vi "ICM Configuration Editor - Copy.vi"(11 "Inside a Program?":bool) -> ()   [LabVIEW 2018]
doc: "ICM Configuration Editor.vi\n\nThis Vi is a graphical configuration editor for ICM.\n\nInstrument Communication Module Version 1.0\nJuly, 2017 Original Code Consulting David Thomson\n www.originalcode.com"
uses:
  Controls/ICM Editor Tab.ctl
  Controls/ICM General Parameters.ctl
  Controls/ICM Config Editor State.ctl
  Controls/ICM Editor Command.ctl
  Scaling/Scaling Def.ctl
  Controls/ICM Config Command.ctl
  Query/Query.lvclass
  Scaling/Scaling.lvclass
  Scaling/Scaling.lvclass/Scaling.ctl
  Query/Query.lvclass/Query.ctl
  Query/Write Cycle Time (ms).vi
  Query/Read Cycle Time (ms).vi
  SubVIs/ICM Editor Stop.vi
  Parser/Parser.lvclass
panel:
  in  "Stop":bool
  in  "File Loaded?":bool
  out "Config File":path
  in  "Tab":T1
  in  "Save As":bool
  in  "Open/New":bool
  in  "Save":bool
  in  "Revert":bool
  in  "ICM General Parameters":T2 {"Time" format="%<%H:%M:%S>t"; "Date" format="%<%Y/%m/%d>T"; "Version" format="%.1g"}
  in  "Save Q":bool
  in  "Revert Q":bool
  in  "Cycle Time (ms)":u32
  in  "Queries":u16(ring) items=["Multiple Queries", "No Query", "Single Query"]
  in  "Bus":u16(ring) items=["Clock Time", "Modbus", "NI Analog", "Serial", "UDP"]
  in  "Parser":u16(ring) items=["General Parser", "Multi Sentence Parser", "No-op Parser", "Time Parser"]
  in  "Delete":bool
  in  "Add":bool
  in  "Instance":u16(ring) items=["(none)", "table", "hello"]
  in  "Save Scaling":bool
  in  "Revert Scaling":bool
  in  "Channel Scalings":i32(listbox)
  in  "Scaling":u16(ring) items=["Lookup Table", "Polynomial"]
  in  "Channel":u16(ring) items=["UTC Time", "Latitiude", "Longititude", "Course Over Ground", "UTS Date of Pos", "Magnetic Variation", "Hour", "Minute", "Second", "Lat", "Long", "Quality", "Satellites", "Horizontal Dilution", "Antenna Height", "Geoidal Height", "Fix Type", "PRN1", "PRN2", "PRN3", "PRN4", "PRN5", "PRN6", "PRN7", "PRN8", "PRN9", "PRN10", "PRN11", "PRN12", "Position Dilution", "Horizontal Dilution", "Vertical Dilution", "Satellites in View", "PRN 1", "Sat Elev 1", "Sat Az 1", "Signal to Noise 1", "PRN 2", "Sat Elev 2", "Sat Az 2", "Signal to Noise 2", "PRN 3", "Sat Elev 3", "Sat Az 3", "Signal to Noise 3", "PRN 4", "Sat Elev 4", "Sat Az 4", "Signal to Noise 4", "Satellites in View", "PRN 5", "Sat Elev 5", "Sat Az 5", "Signal to Noise 5", "PRN 6", "Sat Elev 6", "Sat Az 6", "Signal to Noise 6", "PRN 7", "Sat Elev 7", "Sat Az 7", "Signal to Noise 7", "PRN 8", "Sat Elev 8", "Sat Az 8", "Signal to Noise 8", "Total Number of Satellites", "PRN 9", "Sat Elev 9", "Sat Az 9", "Signal to Noise 9", "PRN 10", "Sat Elev 10", "Sat Az 10", "Signal to Noise 10", "PRN 11", "Sat Elev 11", "Sat Az 11", "Signal to Noise 11", "PRN 12", "Sat Elev 12", "Sat Az 12", "Signal to Noise 12"]
  in  "Output":u16(ring) items=["NI Digital Out"]
  out "Error":errorcluster
  in  "Error Continue":bool
  in  "Error Quit":bool
  in  "Initializer":u16(ring) items=["No Init", "String Init"]
  # "The values for these\nparameters are generally\nset by the ICM system and\nneed not be edited directly."
  # "Entries surrounded by \"***\" are present in the configuration file but\ndo not correspond to existing Channels, Scalings, or Instances."
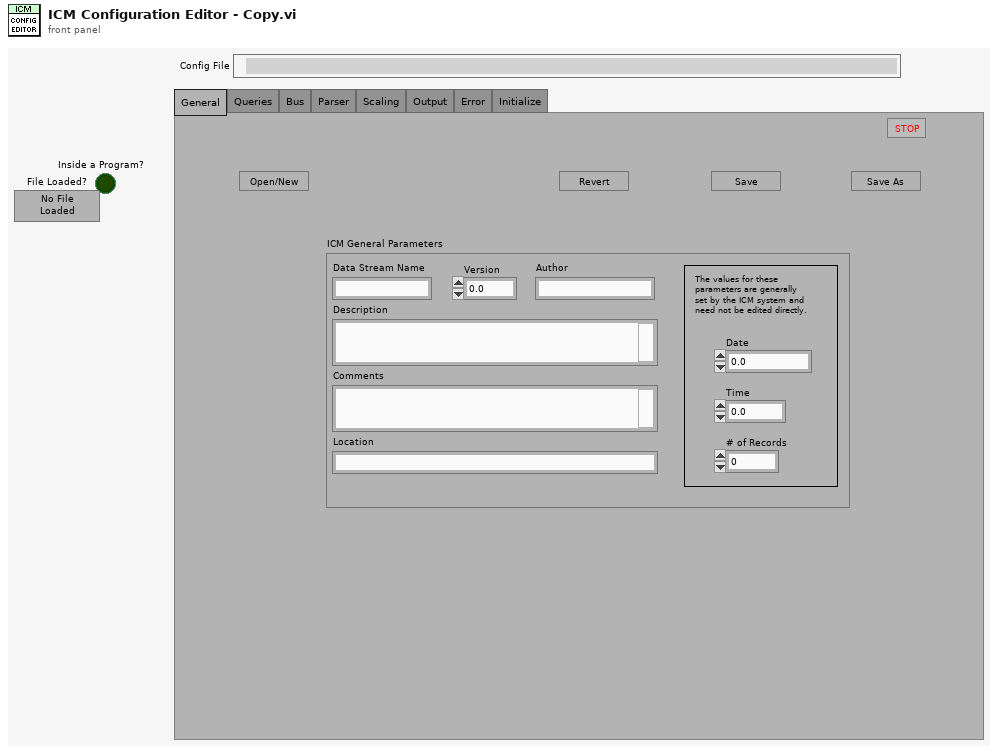
[diagram p1: front panel]
types:
  T1 = typedef "ICM Editor Tab.ctl" = enum32{"General", "Queries", "Bus", "Parser", "Scaling", "Output", "Error", "Initialize"}
  T2 = typedef "ICM General Parameters.ctl" = cluster{"Data Stream Name":string, "Version":sgl, "Author":string, "Description":string, "Comments":string, "Date":dbl, "Time":dbl, "Location":string, "# of Records":i32}
  T3 = typedef "ICM Config Editor State.ctl" = enum16{"Init", "Wait", "Read", "Write", "Load Queries", "Load Bus", "Load Parser", "Display Scaling", "Load Output", "Load Initializer", "Error", "Stop"}
  T4 = typedef "ICM Editor Command.ctl" = enum16{"No-op", "Exit"}
  T5 = typedef "ICM Config Command.ctl" = enum16{"No-op", "Re-Display Sc."}
  T6 = enum8{"Enabled", "Disabled", "Disabled and Grayed Out"}
  T7 = enum32{"Page Enabled", "Page Disabled", "Page Disabled & Grayed"}
  T8 = typedef "Scaling Def.ctl" = cluster{"Channel":string, "Scaling":string, "Instance":string}
  T9 = cluster{"Query.lvclass":refnum<class "Query.lvclass">, "ICM General Parameters":T2, "Output Queue":refnum<queue>, "Init Queue":refnum<queue>, "Config Queue":refnum<queue>, "Scaling Queue":refnum<queue>, "Query Queue":refnum<queue>, "Parser Queue":refnum<queue>, "Bus Queue":refnum<queue>, "Queries Loaded":bool, "Bus Loaded":bool, "Parser Loaded":bool, "Init Loaded":bool, "Output Loaded":bool, "Scaling Loaded":i32, "Instance Loaded":i32, "Scalings":T8[], "Flash?":bool}
  T10 = cluster{"RingText.Text":string, "RingText.Text":string, "RingText.Text":string}
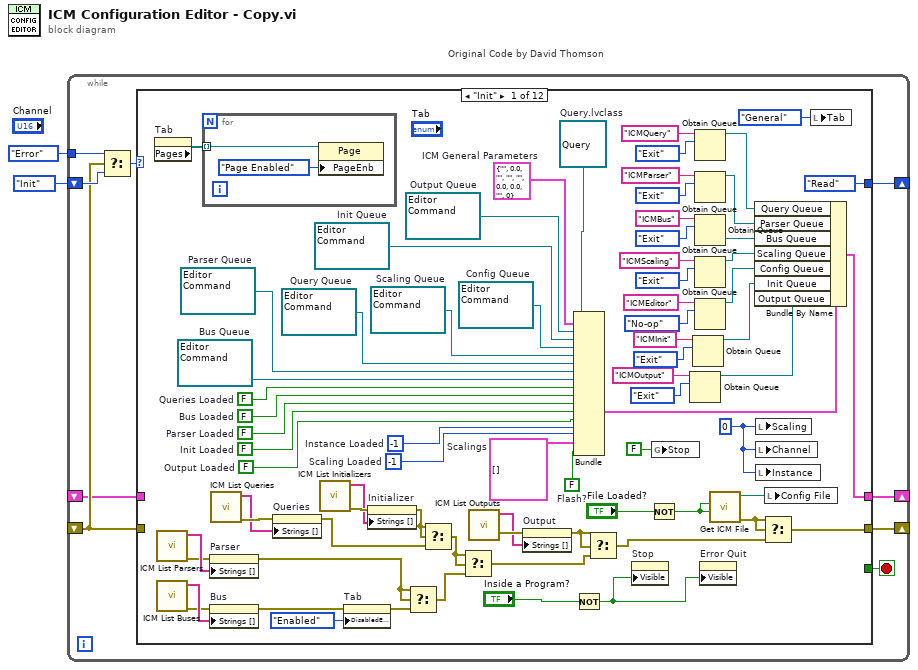
[diagram p0: block diagram]
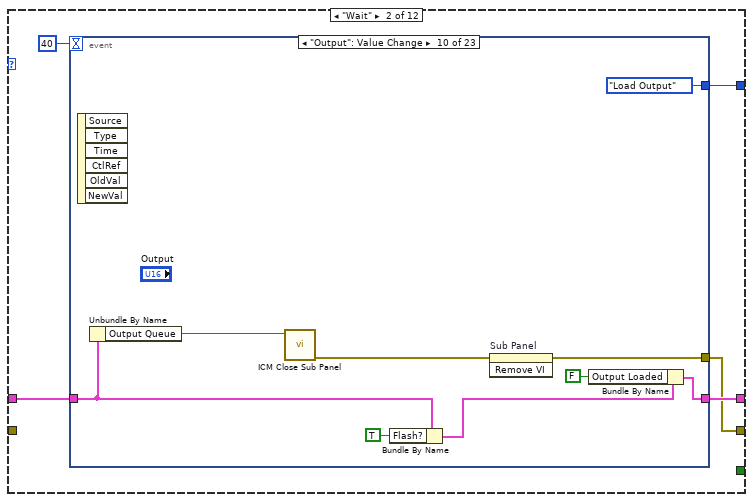
[diagram p2: hidden frame]
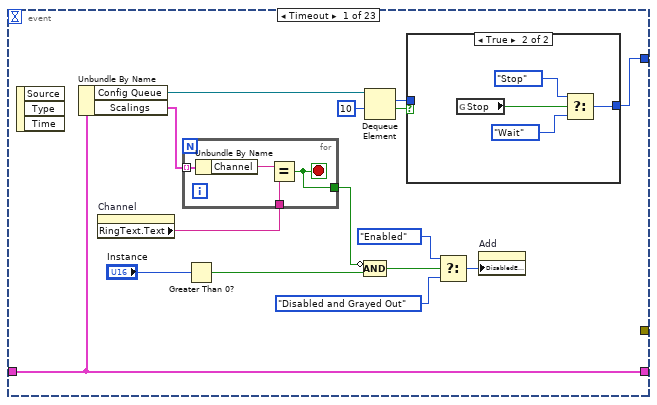
[diagram p3: hidden frame]
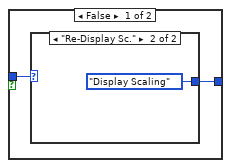
[diagram p4: hidden frame]
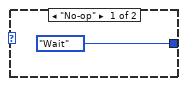
[diagram p5: hidden frame]
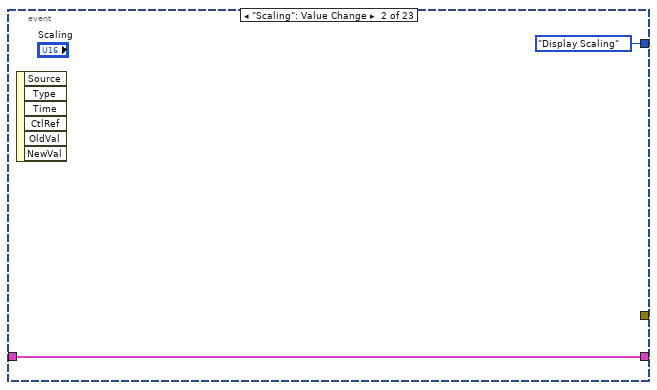
[diagram p6: hidden frame]
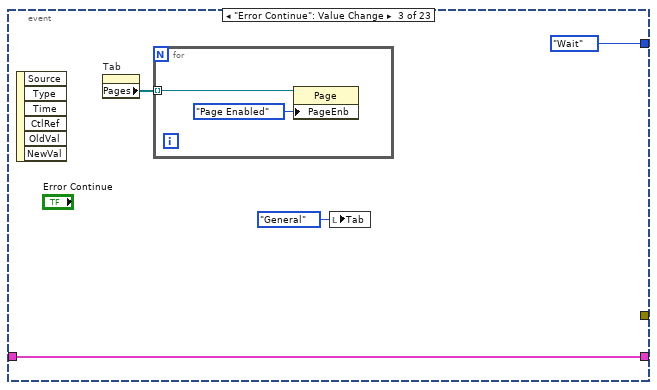
[diagram p7: hidden frame]
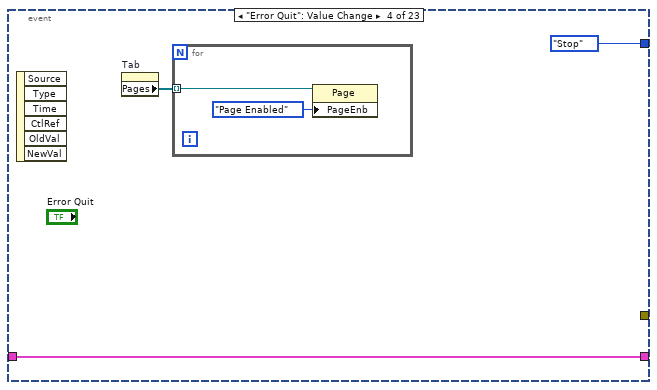
[diagram p8: hidden frame]
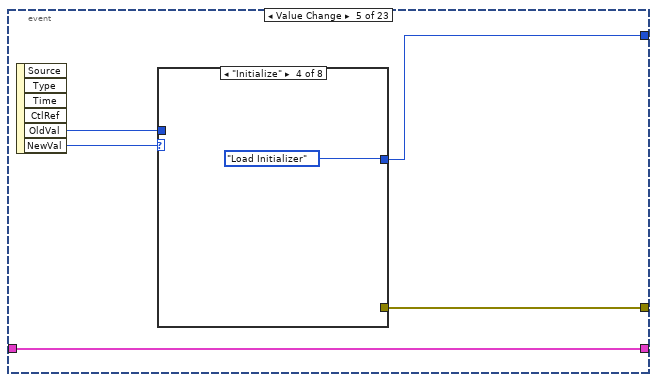
[diagram p9: hidden frame]
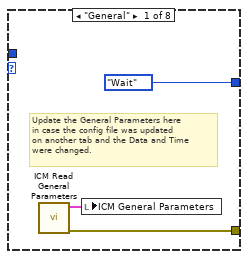
[diagram p10: hidden frame]
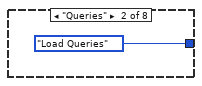
[diagram p11: hidden frame]
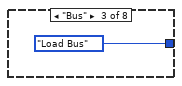
[diagram p12: hidden frame]
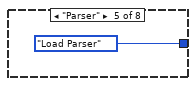
[diagram p13: hidden frame]
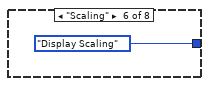
[diagram p14: hidden frame]
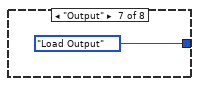
[diagram p15: hidden frame]
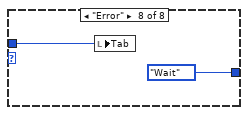
[diagram p16: hidden frame]
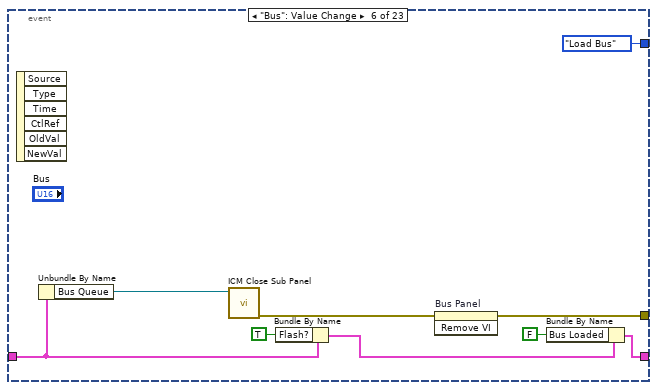
[diagram p17: hidden frame]
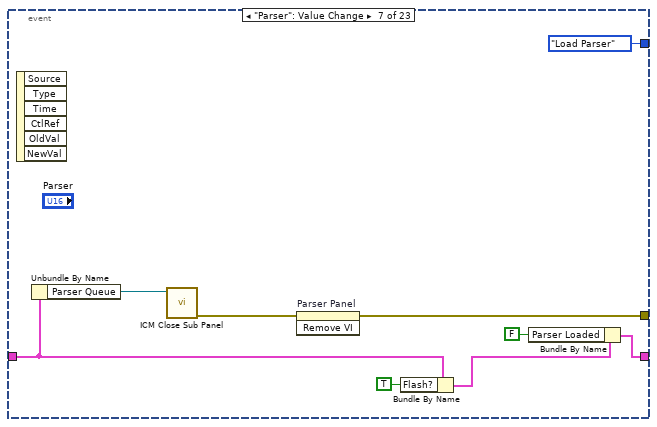
[diagram p18: hidden frame]
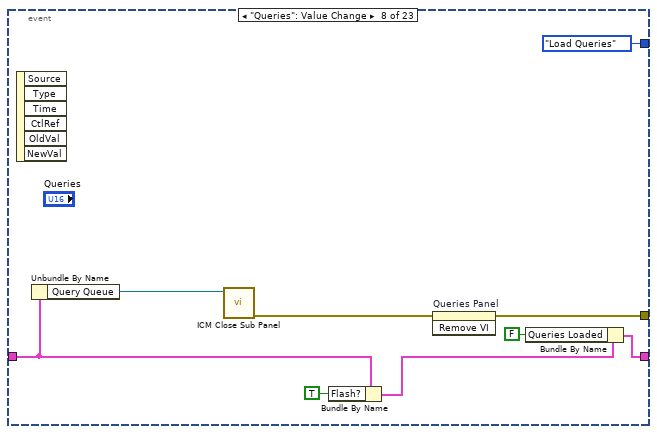
[diagram p19: hidden frame]
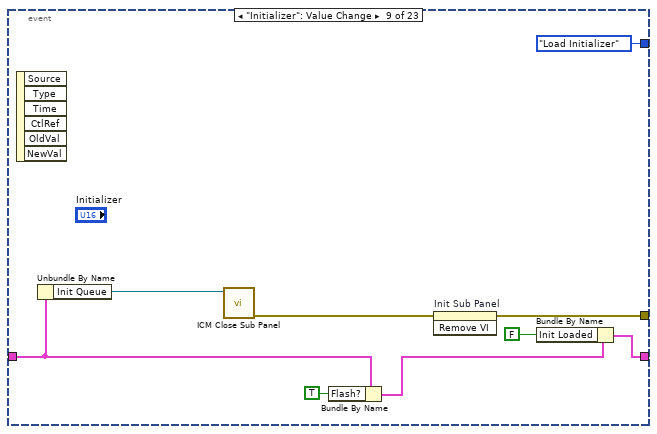
[diagram p20: hidden frame]
diagram:
  n1 = while "Original Code by David Thomson" {
    shift-right: [w5] -> _
    shift-left: ICM_Config_Editor_State."Init" ("Config State") -> [w9]
    shift-right: [w10] -> _
    shift-left: _ -> [w6]
    tunnel: ICM_Config_Editor_State."Error" ("Config State") -> [w7]
    shift-right: [w4] -> _
    shift-left: _ -> [w3]
    stop <- w11 stop-if-true
    n2 = Select(t=w7, s=w6, f=w9) -> (s? t:f=w8:T3)
    n3 = case shown="\"Init\"" w8 {
      tunnel: [_ _ _ _ _ _ _ _ _ _ _ TRUE] -> w11
      tunnel: [w78 w88 w298 w325 w334 w369 w398 w430 w481 _ _ _] -> w10
      tunnel: w6 -> [_ _ _ _ _ _ _ _ _ _ w554 _]
      tunnel: [ICM_Config_Editor_State."Read" ("Config State") w91 ICM_Config_Editor_State."Wait" ("Config State") ICM_Config_Editor_State."Wait" ("Config State") ICM_Config_Editor_State."Wait" ("Config State") ICM_Config_Editor_State."Wait" ("Config State") ICM_Config_Editor_State."Write" ("Config State") ICM_Config_Editor_State."Write" ("Config State") ICM_Config_Editor_State."Wait" ("Config State") ICM_Config_Editor_State."Wait" ("Config State") ICM_Config_Editor_State."Wait" ("Config State") ICM_Config_Editor_State."Stop" ("Config State")] -> w5
      tunnel: [w71 w89 w314 w328 w330 w366 w399 w431 w480 w520 w550 w583] -> w4
      tunnel: w3 -> [_ w90 w316 w328 w336 w367 w400 w432 w467 w520 w550 w583]
      frame "Init" {
        w17 = FALSE  # Output Loaded
        w21 = refnum<queue> refnum items=["No-op", "Exit"]  # Output Queue
        w22 = refnum<queue> refnum items=["No-op", "Exit"]  # Init Queue
        w32 = FALSE  # Init Loaded
        w33 = FALSE  # Flash?
        w42 = refnum<class "Query.lvclass"> refnum  # Query.lvclass
        w31 = refnum<queue> refnum items=["No-op", "Re-Display Sc."]  # Config Queue
        w48 = refnum<queue> refnum items=["No-op", "Exit"]  # Scaling Queue
        w51 = u16 0
        w52 = -1  # Instance Loaded
        w54 = -1  # Scaling Loaded
        w53 = T8[] []  # Scalings
        w59 = refnum<queue> refnum items=["No-op", "Exit"]  # Query Queue
        w67 = refnum<queue> refnum items=["No-op", "Exit"]  # Parser Queue
        w68 = FALSE  # Parser Loaded
        w69 = FALSE  # Bus Loaded
        w70 = FALSE  # Queries Loaded
        w74 = refnum<queue> refnum items=["No-op", "Exit"]  # Bus Queue
        w44 = T2 {"Data Stream Name"="", "Version"=0.0, "Author"="", "Description"="", "Comments"="", "Date"=0.0, "Time"=0.0, "Location"="", "# of Records"=0}  # ICM General Parameters
        n4 = property on="Tab" class="TabCtl (strict)"() -> ("Pages"=w77:refnum<vi>[])  [unwired: 2 in, 2 out]
        n5 = call "ICM List Parsers.vi"() -> ("error out"=w63:errorcluster, "Parsers"=w64:string[])  [unwired: 10 in]
        n6 = call "ICM List Buses.vi"() -> ("error out"=w84:errorcluster, "Buses"=w85:string[])  [unwired: 10 in]
        n7 = for {
          tunnel: w77 -> [w87] mode=indexing
          n8 = property class="Page"(reference=w87, "PageEnb"=T7."Page Enabled" ("Page Enabled State")) -> ()  [unwired: 1 in, 2 out]
        }
        n9 = property on="Parser" class="Ring (strict)"(error in=w63, "Strings []"=w64) -> (error out=w61:errorcluster)  [unwired: 1 in, 1 out]
        n10 = property on="Bus" class="Ring (strict)"(error in=w84, "Strings []"=w85) -> (error out=w82:errorcluster)  [unwired: 1 in, 1 out]
        n11 = call "ICM List Queries.vi"() -> ("error out"=w57:errorcluster, "Queries"=w56:string[])  [unwired: 10 in]
        n12 = property on="Queries" class="Ring (strict)"(error in=w57, "Strings []"=w56) -> (error out=w27:errorcluster)  [unwired: 1 in, 1 out]
        n13 = call "ICM List Initializers.vi"() -> ("error out"=w26:errorcluster, "Initializers"=w25:string[])  [unwired: 10 in]
        n14 = property on="Tab" class="TabCtl (strict)"(error in=w82, "DisabledEnum"=T6."Enabled" ("Disabled")) -> (error out=w62:errorcluster)  [unwired: 1 in, 1 out]
        n15 = property on="Initializer" class="Ring (strict)"(error in=w26, "Strings []"=w25) -> (error out=w24:errorcluster)  [unwired: 1 in, 1 out]
        n16 = Select(t=w61, s=w61, f=w62) -> (s? t:f=w55:errorcluster)
        n17 = Select(t=w24, s=w24, f=w27) -> (s? t:f=w28:errorcluster)
        n18 = Select(t=w28, s=w28, f=w55) -> (s? t:f=w13:errorcluster)
        n19 = call "ICM List Outputs.vi"() -> ("error out"=w16:errorcluster, "Initializers"=w15:string[])  [unwired: 10 in]
        n20 = property on="Output" class="Ring (strict)"(error in=w16, "Strings []"=w15) -> (error out=w12:errorcluster)  [unwired: 1 in, 1 out]
        n21 = Bundle("Query.lvclass"=w42, "ICM General Parameters"=w44, "Output Queue"=w21, "Init Queue"=w22, "Config Queue"=w31, "Scaling Queue"=w48, "Query Queue"=w59, "Parser Queue"=w67, "Bus Queue"=w74, "Queries Loaded"=w70, "Bus Loaded"=w69, "Parser Loaded"=w68, "Init Loaded"=w32, "Output Loaded"=w17, "Scaling Loaded"=w54, "Instance Loaded"=w52, "Scalings"=w53, "Flash?"=w33) -> (w73:T9)  [unwired: 1 in]
        n22 = Not(x="Inside a Program?") -> (.not. x?=w35:bool)
        n23 = Select(t=w12, s=w12, f=w13) -> (s? t:f=w14:errorcluster)
        n24 = property on="Stop" class="Bool"("Visible"=w35) -> ()  [unwired: 2 in, 2 out]
        n25 = Not(x="File Loaded?") -> (.not. x?=w37:bool)
        n26 = global write "ICM Editor Stop.vi" "Stop"(FALSE ("Stop")) -> ()
        n27 = Obtain Queue(name (unnamed)="ICMOutput", element data type=ICM_Editor_Command."Exit" ("Editor Command")) -> (queue out=w18:refnum<queue>)  [unwired: 3 in, 2 out]
        n28 = Obtain Queue(name (unnamed)="ICMInit", element data type=ICM_Editor_Command."Exit" ("Editor Command")) -> (queue out=w23:refnum<queue>)  [unwired: 3 in, 2 out]
        n29 = Obtain Queue(name (unnamed)="ICMQuery", element data type=ICM_Editor_Command."Exit" ("Editor Command")) -> (queue out=w58:refnum<queue>)  [unwired: 3 in, 2 out]
        n30 = Obtain Queue(name (unnamed)="ICMParser", element data type=ICM_Editor_Command."Exit" ("Editor Command")) -> (queue out=w65:refnum<queue>)  [unwired: 3 in, 2 out]
        n31 = Obtain Queue(name (unnamed)="ICMBus", element data type=ICM_Editor_Command."Exit" ("Editor Command")) -> (queue out=w72:refnum<queue>)  [unwired: 3 in, 2 out]
        n32 = Obtain Queue(name (unnamed)="ICMScaling", element data type=ICM_Editor_Command."Exit" ("Editor Command")) -> (queue out=w47:refnum<queue>)  [unwired: 3 in, 2 out]
        n33 = Obtain Queue(name (unnamed)="ICMEditor", element data type=ICM_Config_Command."No-op" ("Editor Command")) -> (queue out=w43:refnum<queue>)  [unwired: 3 in, 2 out]
        n34 = property on="Error Quit" class="Bool"("Visible"=w35) -> ()  [unwired: 2 in, 2 out]
        n35 = call "Get ICM File.vi"("Re-Init?"=w37, "Allow New?"=w37) -> ("error out"=w79:errorcluster, "ICM File"=w76:path)  [unwired: 8 in]
        n36 = Bundle By Name(cluster=w73, "Query Queue"=w58, "Parser Queue"=w65, "Bus Queue"=w72, "Scaling Queue"=w47, "Config Queue"=w43, "Init Queue"=w23, "Output Queue"=w18) -> (w71:T9)
        n37 = local write "Scaling"(w51) -> ()
        n38 = local write "Channel"(w51) -> ()
        n39 = local write "Instance"(w51) -> ()
        n40 = Select(t=w79, s=w79, f=w14) -> (s? t:f=w78:errorcluster)
        n41 = local write "Config File"(w76) -> ()
        n42 = local write "Tab"(ICM_Editor_Tab."General" ("Tab")) -> ()
      }
      frame "Wait" {
        n43 = event shown="[9] \"Output\": Value Change" {
          selector: _ -> [_ _ _ _ _ _ _ _ _ _ _ _ _ _ _ _ _ _ _ _ _ _ _]
          dyn-events: _ -> [_ _ _ _ _ _ _ _ _ _ _ _ _ _ _ _ _ _ _ _ _ _ _]
          timeout: 40 -> [_ _ _ _ _ _ _ _ _ _ _ _ _ _ _ _ _ _ _ _ _ _ _]
          tunnel: [w103 ICM_Config_Editor_State."Display Scaling" ("Config State") ICM_Config_Editor_State."Wait" ("Config State") ICM_Config_Editor_State."Stop" ("Config State") w136 ICM_Config_Editor_State."Load Bus" ("Config State") ICM_Config_Editor_State."Load Parser" ("Config State") ICM_Config_Editor_State."Load Queries" ("Config State") ICM_Config_Editor_State."Load Initializer" ("Config State") ICM_Config_Editor_State."Load Output" ("Config State") ICM_Config_Editor_State."Wait" ("Config State") ICM_Config_Editor_State."Wait" ("Config State") ICM_Config_Editor_State."Write" ("Config State") ICM_Config_Editor_State."Read" ("Config State") w223 ICM_Config_Editor_State."Stop" ("Config State") ICM_Config_Editor_State."Display Scaling" ("Config State") ICM_Config_Editor_State."Display Scaling" ("Config State") ICM_Config_Editor_State."Wait" ("Config State") ICM_Config_Editor_State."Display Scaling" ("Config State") ICM_Config_Editor_State."Wait" ("Config State") ICM_Config_Editor_State."Wait" ("Config State") ICM_Config_Editor_State."Wait" ("Config State")] -> w91
          tunnel: w90 -> [w107 w121 w122 w128 w135 w150 w158 w167 w178 w187 w194 w198 w203 w208 w214 w237 w243 w259 w268 w273 w280 w289 w292]
          tunnel: [w107 w121 w122 w128 w135 w155 w165 w174 w183 w192 w194 w198 w201 w208 w222 w237 w242 w258 w268 w272 w280 w289 w292] -> w89
          tunnel: [_ _ _ _ w134 w156 w163 w172 w177 w185 _ _ _ _ w213 _ _ _ w264 w271 _ w284 w290] -> w88
          event Timeout {
            n44 = event-data() -> ()  [unwired: 1 in, 3 out]
            n45 = Unbundle By Name(w107) -> ("Config Queue"=w106:refnum<queue>, "Scalings"=w101:T8[])
            n46 = property on="Channel" class="Ring (strict)"() -> ("RingText.Text"=w100:string)  [unwired: 2 in, 2 out]
            n47 = for {
              tunnel: w101 -> [w109] mode=indexing
              tunnel: [w111] -> w99
              tunnel: w100 -> [w108]
              stop <- w111 stop-if-true
              n48 = Unbundle By Name(w109) -> ("Channel"=w110:string)
              n49 = Equal?(x=w110, y=w108) -> (x = y?=w111:bool)
            }
            n50 = Greater Than 0?(x="Instance") -> (x > 0?=w97:bool)
            n51 = Compound Arithmetic op=AND(invert w99, w97) -> (w94:bool)
            n52 = Dequeue Element(queue=w106, timeout in ms (-1)=10) -> (element=w102:T5, timed out?=w104:bool)  [unwired: 1 in, 2 out]
            n53 = case shown="True" w104 {
              tunnel: [w112 w119] -> w103
              tunnel: w102 -> [w113 _]
              frame False {
                n54 = case shown="\"Re-Display Sc.\"" w113 {
                  tunnel: [ICM_Config_Editor_State."Wait" ("Config State") ICM_Config_Editor_State."Display Scaling" ("Config State")] -> w112
                  frame "No-op" {
                  }
                  frame "Re-Display Sc." {
                  }
                }
              }
              frame True {
                n55 = global read "ICM Editor Stop.vi" "Stop"() -> (w118:bool)
                n56 = Select(t=ICM_Config_Editor_State."Stop" ("Config State"), s=w118, f=ICM_Config_Editor_State."Wait" ("Config State")) -> (s? t:f=w119:T3)
              }
            }
            n57 = Select(t=T6."Enabled" ("Disabled"), s=w94, f=T6."Disabled and Grayed Out" ("Disabled")) -> (s? t:f=w93:T6)
            n58 = property on="Add" class="Bool"("DisabledEnum"=w93) -> ()  [unwired: 2 in, 2 out]
          }
          event "Scaling": Value Change {
            n59 = event-data() -> ()  [unwired: 1 in, 6 out]
          }
          event "Error Continue": Value Change {
            n60 = event-data() -> ()  [unwired: 1 in, 6 out]
            n61 = property on="Tab" class="TabCtl (strict)"() -> ("Pages"=w123:refnum<vi>[])  [unwired: 2 in, 2 out]
            n62 = for {
              tunnel: w123 -> [w127] mode=indexing
              n63 = property class="Page"(reference=w127, "PageEnb"=T7."Page Enabled" ("Page Enabled State")) -> ()  [unwired: 1 in, 2 out]
            }
            n64 = local write "Tab"(ICM_Editor_Tab."General" ("Tab")) -> ()
          }
          event "Error Quit": Value Change {
            n65 = event-data() -> ()  [unwired: 1 in, 6 out]
            n66 = property on="Tab" class="TabCtl (strict)"() -> ("Pages"=w129:refnum<vi>[])  [unwired: 2 in, 2 out]
            n67 = for {
              tunnel: w129 -> [w132] mode=indexing
              n68 = property class="Page"(reference=w132, "PageEnb"=T7."Page Enabled" ("Page Enabled State")) -> ()  [unwired: 1 in, 2 out]
            }
          }
          event Value Change {
            n69 = event-data() -> ("OldVal"=w133:T1, "NewVal"=w137:T1)  [unwired: 1 in, 4 out]
            n70 = case shown="\"Initialize\"" w137 {
              tunnel: [ICM_Config_Editor_State."Wait" ("Config State") ICM_Config_Editor_State."Load Queries" ("Config State") ICM_Config_Editor_State."Load Bus" ("Config State") ICM_Config_Editor_State."Load Initializer" ("Config State") ICM_Config_Editor_State."Load Parser" ("Config State") ICM_Config_Editor_State."Display Scaling" ("Config State") ICM_Config_Editor_State."Load Output" ("Config State") ICM_Config_Editor_State."Wait" ("Config State")] -> w136
              tunnel: [w138 _ _ _ _ _ _ _] -> w134
              tunnel: w133 -> [_ _ _ _ _ _ _ w147]
              frame "General" {
                # "Update the General Parameters here\nin case the config file was updated\non another tab and the Data and Time\nwere changed."
                n71 = call "ICM Read General Parameters.vi"() -> ("error out"=w138:errorcluster, "ICM General Parameters"=w139:T2)  [unwired: 7 in, 3 out]
                n72 = local write "ICM General Parameters"(w139) -> ()
              }
              frame "Queries" {
              }
              frame "Bus" {
              }
              frame "Initialize" {
              }
              frame "Parser" {
              }
              frame "Scaling" {
              }
              frame "Output" {
              }
              frame "Error" {
                n73 = local write "Tab"(w147) -> ()
              }
            }
          }
          event "Bus": Value Change {
            n74 = event-data() -> ()  [unwired: 1 in, 6 out]
            n75 = Unbundle By Name(w150) -> ("Bus Queue"=w153:refnum<queue>)
            n76 = call "ICM Close Sub Panel.vi"("Queue"=w153) -> ("error out"=w152:errorcluster)  [unwired: 9 in, 1 out]
            n77 = Bundle By Name(cluster=w150, "Flash?"=TRUE) -> (w151:T9)
            n78 = invoke on="Bus Panel" class="SubPnl" method="Remove VI"(error in=w152) -> (error out=w156:errorcluster)  [unwired: 2 in, 2 out]
            n79 = Bundle By Name(cluster=w151, "Bus Loaded"=FALSE) -> (w155:T9)
          }
          event "Parser": Value Change {
            n80 = event-data() -> ()  [unwired: 1 in, 6 out]
            n81 = Unbundle By Name(w158) -> ("Parser Queue"=w162:refnum<queue>)
            n82 = call "ICM Close Sub Panel.vi"("Queue"=w162) -> ("error out"=w161:errorcluster)  [unwired: 9 in, 1 out]
            n83 = invoke on="Parser Panel" class="SubPnl" method="Remove VI"(error in=w161) -> (error out=w163:errorcluster)  [unwired: 2 in, 2 out]
            n84 = Bundle By Name(cluster=w158, "Flash?"=TRUE) -> (w159:T9)
            n85 = Bundle By Name(cluster=w159, "Parser Loaded"=FALSE ("Bus Loaded")) -> (w165:T9)
          }
          event "Queries": Value Change {
            n86 = event-data() -> ()  [unwired: 1 in, 6 out]
            n87 = Unbundle By Name(w167) -> ("Query Queue"=w171:refnum<queue>)
            n88 = call "ICM Close Sub Panel.vi"("Queue"=w171) -> ("error out"=w170:errorcluster)  [unwired: 9 in, 1 out]
            n89 = Bundle By Name(cluster=w167, "Flash?"=TRUE) -> (w168:T9)
            n90 = invoke on="Queries Panel" class="SubPnl" method="Remove VI"(error in=w170) -> (error out=w172:errorcluster)  [unwired: 2 in, 2 out]
            n91 = Bundle By Name(cluster=w168, "Queries Loaded"=FALSE ("Bus Loaded")) -> (w174:T9)
          }
          event "Initializer": Value Change {
            n92 = event-data() -> ()  [unwired: 1 in, 6 out]
            n93 = Unbundle By Name(w178) -> ("Init Queue"=w181:refnum<queue>)
            n94 = call "ICM Close Sub Panel.vi"("Queue"=w181) -> ("error out"=w176:errorcluster)  [unwired: 9 in, 1 out]
            n95 = Bundle By Name(cluster=w178, "Flash?"=TRUE) -> (w179:T9)
            n96 = invoke on="Init Sub Panel" class="SubPnl" method="Remove VI"(error in=w176) -> (error out=w177:errorcluster)  [unwired: 2 in, 2 out]
            n97 = Bundle By Name(cluster=w179, "Init Loaded"=FALSE ("Bus Loaded")) -> (w183:T9)
          }
          event "Output": Value Change {
            n98 = event-data() -> ()  [unwired: 1 in, 6 out]
            n99 = Unbundle By Name(w187) -> ("Output Queue"=w190:refnum<queue>)
            n100 = call "ICM Close Sub Panel.vi"("Queue"=w190) -> ("error out"=w186:errorcluster)  [unwired: 9 in, 1 out]
            n101 = Bundle By Name(cluster=w187, "Flash?"=TRUE) -> (w188:T9)
            n102 = invoke on="Sub Panel" class="SubPnl" method="Remove VI"(error in=w186) -> (error out=w185:errorcluster)  [unwired: 2 in, 2 out]
            n103 = Bundle By Name(cluster=w188, "Output Loaded"=FALSE ("Bus Loaded")) -> (w192:T9)
          }
          event Value Change {
            w196 = TRUE ("Blinking")
            n104 = event-data() -> ()  [unwired: 1 in, 6 out]
            n105 = property on="Revert" class="Bool"("Blinking"=w196) -> ()  [unwired: 2 in, 2 out]
            n106 = property on="Save" class="Bool"("Blinking"=w196) -> ()  [unwired: 2 in, 2 out]
          }
          event "Revert": Value Change {
            w200 = FALSE ("Blinking")
            n107 = event-data() -> ()  [unwired: 1 in, 6 out]
            n108 = Unbundle By Name(w198) -> ("ICM General Parameters"=w197:T2)
            n109 = local write "ICM General Parameters"(w197) -> ()
            n110 = property on="Revert" class="Bool"("Blinking"=w200) -> ()  [unwired: 2 in, 2 out]
            n111 = property on="Save" class="Bool"("Blinking"=w200) -> ()  [unwired: 2 in, 2 out]
          }
          event "Save": Value Change {
            w205 = FALSE ("Blinking")
            n112 = event-data() -> ()  [unwired: 1 in, 6 out]
            n113 = property on="Revert" class="Bool"("Blinking"=w205) -> ()  [unwired: 2 in, 2 out]
            n114 = property on="Save" class="Bool"("Blinking"=w205) -> ()  [unwired: 2 in, 2 out]
            n115 = Bundle By Name(cluster=w203, "ICM General Parameters"="ICM General Parameters") -> (w201:T9)
          }
          event "Open/New": Value Change {
            w206 = TRUE ("Re-Init?")
            n116 = event-data() -> ()  [unwired: 1 in, 6 out]
            n117 = call "Get ICM File.vi"("Re-Init?"=w206, "Allow New?"=w206) -> ("ICM File"=→"Config File":path)  [unwired: 8 in, 1 out]
          }
          event "Save As": Value Change {
            n118 = event-data() -> ()  [unwired: 1 in, 6 out]
            n119 = call "Get ICM File.vi"() -> ("error out"=w216:errorcluster, "ICM File"=w215:path)  [unwired: 10 in]
            n120 = Strip Path(path=w215) -> (stripped path=w221:path)  [unwired: 1 out]
            n121 = call "File Dialog"("start path"=w221, "prompt"="Name the new configuration file:" ("pattern label"), "error in"=w216, "pattern (all files)"=".icm", "pattern label"="ICM Configuraiton File") -> ("selected path"=w217:path, "cancelled"=w211:bool, "error out"=w212:errorcluster)  [unwired: 7 in, 1 out]
            n122 = Compound Arithmetic op=AND(invert w211, invert w212) -> (w210:bool)
            n123 = case shown="True" w210 {
              tunnel: [ICM_Config_Editor_State."Wait" ("Config State") ICM_Config_Editor_State."Write" ("Config State")] -> w223
              tunnel: [w225 w227] -> w222
              tunnel: w217 -> [_ w232]
              tunnel: w215 -> [_ w234]
              tunnel: w214 -> [w225 w228]
              tunnel: [_ w229] -> w213
              frame False {
              }
              frame True {
                w235 = FALSE ("Blinking")
                n124 = Copy(9:TRUE ("overwrite (F)"), 10:w232, 11:w234) -> (0:w230:errorcluster)  [unwired: 2 in, 2 out]
                n125 = call "Get ICM File.vi"("ICM File In"=w232) -> ("error out"=w231:errorcluster)  [unwired: 9 in, 1 out]
                n126 = Select(t=w231, s=w231, f=w230) -> (s? t:f=w229:errorcluster)
                n127 = local read "ICM General Parameters"() -> (w226:T2)
                n128 = Bundle By Name(cluster=w228, "ICM General Parameters"=w226) -> (w227:T9)
                n129 = property on="Revert" class="Bool"("Blinking"=w235) -> ()  [unwired: 2 in, 2 out]
                n130 = property on="Save" class="Bool"("Blinking"=w235) -> ()  [unwired: 2 in, 2 out]
              }
            }
          }
          event "Stop": Value Change {
            n131 = event-data() -> ()  [unwired: 1 in, 6 out]
          }
          event "Add": Value Change {
            n132 = event-data() -> ()  [unwired: 1 in, 6 out]
            n133 = property on="Channel" class="Ring (strict)"() -> ("RingText.Text"=w241:string)  [unwired: 2 in, 2 out]
            n134 = property on="Scaling" class="Ring (strict)"() -> ("RingText.Text"=w247:string)  [unwired: 2 in, 2 out]
            n135 = property on="Instance" class="Ring (strict)"() -> ("RingText.Text"=w246:string)  [unwired: 2 in, 2 out]
            n136 = Unbundle By Name(w243) -> ("Scalings"=w240:T8[])
            n137 = Bundle("RingText.Text"=w241, "RingText.Text"=w247, "RingText.Text"=w246) -> (w245:T10)  [unwired: 1 in]
            n138 = for {
              tunnel: w241 -> [w250]
              tunnel: w240 -> [w252] mode=indexing
              tunnel: [w249] -> w239
              stop <- w249 stop-if-true
              n139 = Unbundle By Name(w252) -> ("Channel"=w251:string)
              n140 = Equal?(x=w250, y=w251) -> (x = y?=w249:bool)
            }
            n141 = case shown="False" w239 {
              tunnel: w245 -> [w255 _]
              tunnel: w240 -> [w254 w256]
              tunnel: [w253 w256] -> w244
              frame False {
                n142 = Build Array (concatenate)(w255, w254) -> (w253:T8[])
              }
              frame True {
              }
            }
            n143 = Bundle By Name(cluster=w243, "Scalings"=w244) -> (w242:T9)
          }
          event "Delete": Value Change {
            n144 = event-data() -> ()  [unwired: 1 in, 6 out]
            n145 = Unbundle By Name(w259) -> ("Scalings"=w262:T8[])
            n146 = Delete From Array(array=w262, length=1, index="Channel Scalings") -> (array with subset deleted=w260:T8[])  [unwired: 1 out]
            n147 = Bundle By Name(cluster=w259, "Scalings"=w260) -> (w258:T9)
          }
          event "Save Scaling": Value Change {
            n148 = event-data() -> ()  [unwired: 1 in, 6 out]
            n149 = Unbundle By Name(w268) -> ("Scalings"=w267:T8[])
            n150 = call "Write Scalings.vi"("Scalings"=w267, "Scaling in"=refnum<class "Scaling.lvclass"> refnum ("Scaling.lvclass")) -> ("error out"=w265:errorcluster, "Scaling out"=w266:refnum<class "Scaling.lvclass">)  [unwired: 8 in]
            n151 = call-dynamic "Write Config.vi"("error in (no error)"=w265, "Scaling in"=w266) -> ("error out"=w264:errorcluster)  [unwired: 8 in, 1 out]
          }
          event "Revert Scaling": Value Change {
            n152 = event-data() -> ()  [unwired: 1 in, 6 out]
            n153 = call-dynamic "Read Config.vi"("Scaling in"=refnum<class "Scaling.lvclass"> refnum ("Scaling.lvclass")) -> ("error out"=w276:errorcluster, "Scaling out"=w275:refnum<class "Scaling.lvclass">)  [unwired: 9 in]
            n154 = call "Read Scalings.vi"("error in (no error)"=w276, "Scaling in"=w275) -> ("error out"=w271:errorcluster, "Scalings"=w274:T8[])  [unwired: 7 in, 1 out]
            n155 = Bundle By Name(cluster=w273, "Scalings"=w274) -> (w272:T9)
          }
          event "Cycle Time (ms)": Value Change {
            w279 = TRUE ("Blinking")
            n156 = event-data() -> ()  [unwired: 1 in, 6 out]
            n157 = property on="Revert Q" class="Bool"("Blinking"=w279) -> ()  [unwired: 2 in, 2 out]
            n158 = property on="Save Q" class="Bool"("Blinking"=w279) -> ()  [unwired: 2 in, 2 out]
          }
          event "Save Q": Value Change {
            w282 = FALSE ("Blinking")
            n159 = event-data() -> ()  [unwired: 1 in, 6 out]
            n160 = Unbundle By Name(w289) -> ("Query.lvclass"=w288:refnum<class "Query.lvclass">)
            n161 = property class="Query.lvclass"(reference=w288, "Properties:Cycle Time (ms)"="Cycle Time (ms)") -> (reference out=w286:refnum<class "Query.lvclass">, error out=w285:errorcluster)  [unwired: 1 in]
            n162 = call-dynamic "Write Config.vi"("error in (no error)"=w285, "Query in"=w286) -> ("error out"=w284:errorcluster)  [unwired: 8 in, 1 out]
            n163 = property on="Revert Q" class="Bool"("Blinking"=w282) -> ()  [unwired: 2 in, 2 out]
            n164 = property on="Save Q" class="Bool"("Blinking"=w282) -> ()  [unwired: 2 in, 2 out]
          }
          event "Revert Q": Value Change {
            w295 = FALSE ("Blinking")
            n165 = event-data() -> ()  [unwired: 1 in, 6 out]
            n166 = property on="Revert Q" class="Bool"("Blinking"=w295) -> ()  [unwired: 2 in, 2 out]
            n167 = property on="Save Q" class="Bool"("Blinking"=w295) -> ()  [unwired: 2 in, 2 out]
            n168 = Unbundle By Name(w292) -> ("Query.lvclass"=w293:refnum<class "Query.lvclass">)
            n169 = property class="Query.lvclass"(reference=w293) -> (error out=w290:errorcluster, "Properties:Cycle Time (ms)"=w291:u32)  [unwired: 1 in, 1 out]
            n170 = local write "Cycle Time (ms)"(w291) -> ()
          }
        }
      }
      frame "Read" {
        n171 = property on="Queries" class="Ring (strict)"() -> ("Strings []"=w304:string[])  [unwired: 2 in, 2 out]
        n172 = property on="Bus" class="Ring (strict)"() -> ("Strings []"=w321:string[])  [unwired: 2 in, 2 out]
        n173 = property on="Parser" class="Ring (strict)"() -> ("Strings []"=w308:string[])  [unwired: 2 in, 2 out]
        n174 = call "ICM Read General Parameters.vi"() -> ("error out"=w301:errorcluster, "Parser"=w310:string, "Bus"=w322:string, "ICM General Parameters"=w315:T2, "Query"=w302:string)  [unwired: 7 in]
        n175 = Search 1D Array(1D array=w321, element=w322) -> (index of element=w319:i32)  [unwired: 1 in]
        n176 = Search 1D Array(1D array=w308, element=w310) -> (index of element=w312:i32)  [unwired: 1 in]
        n177 = Search 1D Array(1D array=w304, element=w302) -> (index of element=w307:i32)  [unwired: 1 in]
        n178 = Less Than 0?(x=w319) -> (x < 0?=w320:bool)
        n179 = Less Than 0?(x=w312) -> (x < 0?=w311:bool)
        n180 = Less Than 0?(x=w307) -> (x < 0?=w306:bool)
        n181 = call-dynamic "Read Config.vi"("error in (no error)"=w301, "Scaling in"=refnum<class "Scaling.lvclass"> refnum ("Scaling.lvclass")) -> ("error out"=w299:errorcluster, "Scaling out"=w297:refnum<class "Scaling.lvclass">)  [unwired: 8 in]
        n182 = Select(t=0, s=w320, f=w319) -> (s? t:f=w317:i32)
        n183 = Select(t=0, s=w311, f=w312) -> (s? t:f=w309:i32)
        n184 = Select(t=0, s=w306, f=w307) -> (s? t:f=w303:i32)
        n185 = local write "Queries"(w303) -> ()
        n186 = local write "Bus"(w317) -> ()
        n187 = local write "Parser"(w309) -> ()
        n188 = call "Read Scalings.vi"("error in (no error)"=w299, "Scaling in"=w297) -> ("error out"=w298:errorcluster, "Scalings"=w296:T8[])  [unwired: 7 in, 1 out]
        n189 = local write "ICM General Parameters"(w315) -> ()
        n190 = Bundle By Name(cluster=w316, "ICM General Parameters"=w315, "Scalings"=w296) -> (w314:T9)
      }
      frame "Write" {
        n191 = Unbundle By Name(w328) -> ("ICM General Parameters"=w327:T2)
        n192 = call "ICM Write General Parameters.vi"("ICM General Parameters"=w327) -> ("error out"=w326:errorcluster)  [unwired: 10 in]
        n193 = call "ICM Update Date and Time.vi"("error in (no error)"=w326) -> ("error out"=w325:errorcluster, "output cluster"=w324:T2)  [unwired: 9 in]
        n194 = local write "ICM General Parameters"(w324) -> ()
      }
      frame "Load Queries" {
        n195 = Unbundle By Name(w336) -> ("Query.lvclass"=w335:refnum<class "Query.lvclass">, "Queries Loaded"=w337:bool)
        n196 = call-dynamic "Read Config.vi"("Query in"=w335) -> ("error out"=w332:errorcluster, "Query out"=w333:refnum<class "Query.lvclass">)  [unwired: 9 in]
        n197 = case shown="False" w337 {
          tunnel: [w350 _] -> w334
          tunnel: w336 -> [w339 w365]
          tunnel: [w351 w365] -> w330
          frame False {
            n198 = call "ICM Queries Path.vi"() -> ("error out"=w345:errorcluster, "ICM Queries Path"=w359:path)  [unwired: 10 in]
            n199 = property on="Queries" class="Ring (strict)"(error in=w345) -> (error out=w346:errorcluster, "RingText.Text"=w347:string)  [unwired: 1 in, 1 out]
            n200 = Unbundle By Name(w339) -> ("Flash?"=w344:bool)
            n201 = Build Path(base path=w359, name or relative path=w347) -> (appended path=w358:path)
            n202 = Build Path(base path=w358, name or relative path="Edit Config.vi") -> (appended path=w356:path)
            n203 = Open VI Reference(vi path=w356, error in (no error)=w346) -> (vi reference=w342:refnum<vi>, error out=w355:errorcluster)  [unwired: 4 in]
            n204 = case shown="True" w344 {
              tunnel: w342 -> [w360 w362]
              tunnel: [w360 w361] -> w341
              frame False {
              }
              frame True {
                n205 = invoke class="VI" method="Ctrl Val.Set"(reference=w362, "Control Name"="Flash Save", "Value"=TRUE ("Bus Loaded")) -> (reference out=w361:refnum<vi>)  [unwired: 2 in, 4 out]
              }
            }
            n206 = Bundle By Name(cluster=w339, "Flash?"=FALSE) -> (w340:T9)
            n207 = invoke class="VI" method="Run VI"(reference=w341, error in=w355, "Wait until done"=FALSE ("Wait Until Done"), "Auto Dispose Ref"=TRUE ("Auto Dispose Reference")) -> (reference out=w348:refnum<vi>, error out=w349:errorcluster)  [unwired: 1 in, 3 out]
            n208 = Bundle By Name(cluster=w340, "Queries Loaded"=TRUE ("Bus Loaded")) -> (w351:T9)
            n209 = invoke on="Queries Panel" class="SubPnl" method="Insert VI"(error in=w349, "VI Ref"=w348) -> (error out=w350:errorcluster)  [unwired: 2 in, 3 out]
          }
          frame True {
          }
        }
        n210 = property class="Query.lvclass"(reference=w333, error in=w332) -> ("Properties:Cycle Time (ms)"=w331:u32)  [unwired: 2 out]
        n211 = local write "Cycle Time (ms)"(w331) -> ()
      }
      frame "Load Bus" {
        n212 = Unbundle By Name(w367) -> ("Bus Loaded"=w368:bool)
        n213 = case shown="False" w368 {
          tunnel: [w379 _] -> w369
          tunnel: w367 -> [w372 w397]
          tunnel: [w377 w397] -> w366
          frame False {
            n214 = call "ICM Buses Path.vi"() -> ("error out"=w391:errorcluster, "ICM Buses Path"=w390:path)  [unwired: 10 in]
            n215 = property on="Bus" class="Ring (strict)"(error in=w391) -> (error out=w384:errorcluster, "RingText.Text"=w389:string)  [unwired: 1 in, 1 out]
            n216 = Build Path(base path=w390, name or relative path=w389) -> (appended path=w388:path)
            n217 = Unbundle By Name(w372) -> ("Flash?"=w374:bool)
            n218 = Build Path(base path=w388, name or relative path="Edit Config.vi") -> (appended path=w386:path)
            n219 = Open VI Reference(vi path=w386, error in (no error)=w384) -> (vi reference=w376:refnum<vi>, error out=w385:errorcluster)  [unwired: 4 in]
            n220 = case shown="True" w374 {
              tunnel: w376 -> [w392 w394]
              tunnel: [w392 w393] -> w375
              frame False {
              }
              frame True {
                n221 = invoke class="VI" method="Ctrl Val.Set"(reference=w394, "Control Name"="Flash Save", "Value"=TRUE ("Bus Loaded")) -> (reference out=w393:refnum<vi>)  [unwired: 2 in, 4 out]
              }
            }
            n222 = Bundle By Name(cluster=w372, "Flash?"=FALSE) -> (w373:T9)
            n223 = invoke class="VI" method="Run VI"(reference=w375, error in=w385, "Wait until done"=FALSE ("Wait Until Done"), "Auto Dispose Ref"=TRUE ("Auto Dispose Reference")) -> (reference out=w380:refnum<vi>, error out=w381:errorcluster)  [unwired: 1 in, 3 out]
            n224 = Bundle By Name(cluster=w373, "Bus Loaded"=TRUE) -> (w377:T9)
            n225 = invoke on="Bus Panel" class="SubPnl" method="Insert VI"(error in=w381, "VI Ref"=w380) -> (error out=w379:errorcluster)  [unwired: 2 in, 3 out]
          }
          frame True {
          }
        }
      }
      frame "Load Parser" {
        n226 = Unbundle By Name(w400) -> ("Parser Loaded"=w401:bool)
        n227 = case shown="False" w401 {
          tunnel: [w414 _] -> w398
          tunnel: w400 -> [w406 w429]
          tunnel: [w415 w429] -> w399
          frame False {
            n228 = call "ICM Parsers Path.vi"() -> ("error out"=w410:errorcluster, "ICM Parsers Path"=w423:path)  [unwired: 10 in]
            n229 = property on="Parser" class="Ring (strict)"(error in=w410) -> (error out=w409:errorcluster, "RingText.Text"=w411:string)  [unwired: 1 in, 1 out]
            n230 = Unbundle By Name(w406) -> ("Flash?"=w408:bool)
            n231 = Build Path(base path=w423, name or relative path=w411) -> (appended path=w422:path)
            n232 = Build Path(base path=w422, name or relative path="Edit Config.vi") -> (appended path=w420:path)
            n233 = Open VI Reference(vi path=w420, error in (no error)=w409) -> (vi reference=w404:refnum<vi>, error out=w419:errorcluster)  [unwired: 4 in]
            n234 = case shown="True" w408 {
              tunnel: w404 -> [w424 w426]
              tunnel: [w424 w425] -> w403
              frame False {
              }
              frame True {
                n235 = invoke class="VI" method="Ctrl Val.Set"(reference=w426, "Control Name"="Flash Save", "Value"=TRUE ("Bus Loaded")) -> (reference out=w425:refnum<vi>)  [unwired: 2 in, 4 out]
              }
            }
            n236 = Bundle By Name(cluster=w406, "Flash?"=FALSE) -> (w405:T9)
            n237 = invoke class="VI" method="Run VI"(reference=w403, error in=w419, "Wait until done"=FALSE ("Wait Until Done"), "Auto Dispose Ref"=TRUE ("Auto Dispose Reference")) -> (reference out=w412:refnum<vi>, error out=w413:errorcluster)  [unwired: 1 in, 3 out]
            n238 = Bundle By Name(cluster=w405, "Parser Loaded"=TRUE ("Bus Loaded")) -> (w415:T9)
            n239 = invoke on="Parser Panel" class="SubPnl" method="Insert VI"(error in=w413, "VI Ref"=w412) -> (error out=w414:errorcluster)  [unwired: 2 in, 3 out]
          }
          frame True {
          }
        }
      }
      frame "Load Initializer" {
        n240 = Unbundle By Name(w432) -> ("Init Loaded"=w433:bool)
        n241 = case shown="False" w433 {
          tunnel: [w438 _] -> w430
          tunnel: w432 -> [w444 w461]
          tunnel: [w447 w461] -> w431
          frame False {
            n242 = call "ICM Initializers Path.vi"() -> ("error out"=w437:errorcluster, "ICM Queries Path"=w455:path)  [unwired: 10 in]
            n243 = property on="Initializer" class="Ring (strict)"(error in=w437) -> (error out=w436:errorcluster, "RingText.Text"=w435:string)  [unwired: 1 in, 1 out]
            n244 = Unbundle By Name(w444) -> ("Flash?"=w446:bool)
            n245 = Build Path(base path=w455, name or relative path=w435) -> (appended path=w454:path)
            n246 = Build Path(base path=w454, name or relative path="Edit Config.vi") -> (appended path=w452:path)
            n247 = Open VI Reference(vi path=w452, error in (no error)=w436) -> (vi reference=w442:refnum<vi>, error out=w451:errorcluster)  [unwired: 4 in]
            n248 = case shown="True" w446 {
              tunnel: w442 -> [w456 w458]
              tunnel: [w456 w457] -> w441
              frame False {
              }
              frame True {
                n249 = invoke class="VI" method="Ctrl Val.Set"(reference=w458, "Control Name"="Flash Save", "Value"=TRUE ("Bus Loaded")) -> (reference out=w457:refnum<vi>)  [unwired: 2 in, 4 out]
              }
            }
            n250 = Bundle By Name(cluster=w444, "Flash?"=FALSE) -> (w443:T9)
            n251 = invoke class="VI" method="Run VI"(reference=w441, error in=w451, "Wait until done"=FALSE ("Wait Until Done"), "Auto Dispose Ref"=TRUE ("Auto Dispose Reference")) -> (reference out=w440:refnum<vi>, error out=w439:errorcluster)  [unwired: 1 in, 3 out]
            n252 = Bundle By Name(cluster=w443, "Init Loaded"=TRUE ("Bus Loaded")) -> (w447:T9)
            n253 = invoke on="Init Sub Panel" class="SubPnl" method="Insert VI"(error in=w439, "VI Ref"=w440) -> (error out=w438:errorcluster)  [unwired: 2 in, 3 out]
          }
          frame True {
          }
        }
      }
      frame "Display Scaling" {
        n254 = Unbundle By Name(w467) -> ("Scaling Loaded"=w462:i32, "Instance Loaded"=w472:i32, "Scaling Queue"=w471:refnum<queue>)
        n255 = Unbundle By Name(w467) -> ("Scalings"=w466:T8[])
        n256 = local read "Instance"() -> (w478:u16)
        n257 = local read "Scaling"() -> (w479:u16)
        n258 = call "ICM List Scalings.vi"() -> ("error out"=w488:errorcluster, "Scalings"=w465:string[])  [unwired: 10 in]
        n259 = To Long Integer(number=w479) -> (32bit integer=w475:i32)
        n260 = To Long Integer(number=w478) -> (32bit integer=w473:i32)
        n261 = property on="Scaling" class="Ring (strict)"(error in=w488, "Strings []"=w465) -> (error out=w487:errorcluster)  [unwired: 1 in, 1 out]
        n262 = Not Equal?(x=w473, y=w472) -> (x != y?=w476:bool)
        n263 = Not Equal?(x=w475, y=w462) -> (x != y?=w474:bool)
        n264 = Or(x=w476, y=w474) -> (x .or. y?=w477:bool)
        n265 = call "ICM Open Parser.vi"("error in (no error)"=w487) -> ("error out"=w490:errorcluster, "Parser out"=w491:refnum<class "Parser.lvclass">)  [unwired: 9 in]
        n266 = call-dynamic "Read Enabled Channels.vi"("error in (no error)"=w490, "Parser in"=w491) -> ("error out"=w489:errorcluster, "Enabled Channels"=w464:string[])  [unwired: 7 in, 1 out]
        n267 = property on="Channel" class="Ring (strict)"(error in=w489, "Strings []"=w464) -> (error out=w486:errorcluster)  [unwired: 1 in, 1 out]
        n268 = call "ICM List Scaling Instances.vi"("error in (no error)"=w486, "Scalings"=w465) -> ("error out"=w485:errorcluster, "Instances"=w463:cluster{"Instances":string[]}[])  [unwired: 8 in]
        n269 = call "ICM VI Template.vi"("Instances"=w463, "Scalings"=w465, "Channels"=w464, "Scalings In"=w466) -> ("Table"=w468:string[][])  [unwired: 7 in]
        n270 = property on="Channel Scalings" class="MCListbox (strict)"("ItemNames"=w468) -> ()  [unwired: 2 in, 2 out]
        n271 = local read "Scaling"() -> (w483:u16)
        n272 = Index Array(array=w463, index=w483) -> (element=w484:cluster{"Instances":string[]})
        n273 = Unbundle(w484) -> ("Instances"=w469:string[])
        n274 = case shown="True" w477 {
          tunnel: [_ w504] -> w482
          tunnel: w467 -> [w493 w503]
          tunnel: [w493 w502] -> w480
          tunnel: w475 -> [_ w501]
          tunnel: w473 -> [_ w500]
          tunnel: w471 -> [_ w499]
          tunnel: w469 -> [_ _]
          tunnel: w462 -> [_ w496]
          frame False {
          }
          frame True {
            n275 = flat-sequence {
              tunnel: [w519] -> w515
              tunnel: [w518] -> w507
              tunnel: w497 -> [_]
              frame #0 {
                n276 = call "ICM Scalings Path.vi"() -> ("error out"=w518:errorcluster, "ICM Scalings Path"=w519:path)  [unwired: 10 in]
              }
            }
            n277 = Bundle By Name(cluster=w503, "Instance Loaded"=w500, "Scaling Loaded"=w501) -> (w502:T9)
            n278 = case shown="0.." w496 {
              tunnel: w499 -> [_ w517]
              tunnel: [_ w516] -> w498
              frame ..-1 {
              }
              frame 0.. {
                n279 = call "ICM Close Sub Panel.vi"("Queue"=w517) -> ("error out"=w516:errorcluster)  [unwired: 9 in, 1 out]
              }
            }
            n280 = property on="Scaling" class="Ring (strict)"(error in=w507) -> (error out=w509:errorcluster, "RingText.Text"=w508:string)  [unwired: 1 in, 1 out]
            n281 = invoke on="Scaling" class="SubPnl" method="Remove VI"(error in=w498) -> (error out=w497:errorcluster)  [unwired: 2 in, 2 out]
            n282 = Build Path(base path=w515, name or relative path=w508) -> (appended path=w514:path)
            n283 = Build Path(base path=w514, name or relative path="Edit Config.vi") -> (appended path=w512:path)
            n284 = Open VI Reference(vi path=w512, error in (no error)=w509) -> (vi reference=w494:refnum<vi>, error out=w495:errorcluster)  [unwired: 4 in]
            n285 = invoke class="VI" method="Run VI"(reference=w494, error in=w495, "Wait until done"=FALSE ("Wait Until Done"), "Auto Dispose Ref"=TRUE ("Auto Dispose Reference")) -> (reference out=w506:refnum<vi>, error out=w505:errorcluster)  [unwired: 1 in, 3 out]
            n286 = invoke on="Scaling" class="SubPnl" method="Insert VI"(error in=w505, "VI Ref"=w506) -> (error out=w504:errorcluster)  [unwired: 2 in, 3 out]
          }
        }
        n287 = property on="Instance" class="Ring (strict)"(error in=w485, "Strings []"=w469) -> (error out=w470:errorcluster)  [unwired: 1 in, 1 out]
        n288 = Select(t=w470, s=w470, f=w482) -> (s? t:f=w481:errorcluster)
      }
      frame "Load Output" {
        n289 = Unbundle By Name(w520) -> ("Output Loaded"=w521:bool)
        n290 = case shown="False" w521 {
          tunnel: [w524 _] -> _
          tunnel: w520 -> [w530 w549]
          tunnel: [w535 w549] -> _
          frame False {
            n291 = call "ICM Outputs Path.vi"() -> ("error out"=w527:errorcluster, "ICM Queries Path"=w543:path)  [unwired: 10 in]
            n292 = property on="Output" class="Ring (strict)"(error in=w527) -> (error out=w528:errorcluster, "RingText.Text"=w526:string)  [unwired: 1 in, 1 out]
            n293 = Unbundle By Name(w530) -> ("Flash?"=w532:bool)
            n294 = Build Path(base path=w543, name or relative path=w526) -> (appended path=w542:path)
            n295 = Build Path(base path=w542, name or relative path="Edit Config.vi") -> (appended path=w540:path)
            n296 = Open VI Reference(vi path=w540, error in (no error)=w528) -> (vi reference=w534:refnum<vi>, error out=w539:errorcluster)  [unwired: 4 in]
            n297 = case shown="True" w532 {
              tunnel: w534 -> [w544 w546]
              tunnel: [w544 w545] -> w533
              frame False {
              }
              frame True {
                n298 = invoke class="VI" method="Ctrl Val.Set"(reference=w546, "Control Name"="Flash Save", "Value"=TRUE ("Bus Loaded")) -> (reference out=w545:refnum<vi>)  [unwired: 2 in, 4 out]
              }
            }
            n299 = Bundle By Name(cluster=w530, "Flash?"=FALSE) -> (w531:T9)
            n300 = invoke class="VI" method="Run VI"(reference=w533, error in=w539, "Wait until done"=FALSE ("Wait Until Done"), "Auto Dispose Ref"=TRUE ("Auto Dispose Reference")) -> (reference out=w525:refnum<vi>, error out=w523:errorcluster)  [unwired: 1 in, 3 out]
            n301 = Bundle By Name(cluster=w531, "Output Loaded"=TRUE ("Bus Loaded")) -> (w535:T9)
            n302 = invoke on="Sub Panel" class="SubPnl" method="Insert VI"(error in=w523, "VI Ref"=w525) -> (error out=w524:errorcluster)  [unwired: 2 in, 3 out]
          }
          frame True {
          }
        }
      }
      frame "Error" {
        n303 = property on="Tab" class="TabCtl (strict)"() -> ("Pages"=w551:refnum<vi>[])  [unwired: 2 in, 2 out]
        n304 = local write "Tab"(ICM_Editor_Tab."Error" ("Tab")) -> ()
        n305 = for {
          tunnel: w551 -> [w562] mode=indexing
          n306 = property class="Page"(reference=w562) -> (reference out=w559:refnum<vi>, "PageLabel"=w561:string)  [unwired: 1 in, 1 out]
          n307 = Equal?(x=w561, y="Error") -> (x = y?=w556:bool)
          n308 = Select(t=T7."Page Enabled" ("Page Enabled State"), s=w556, f=T7."Page Disabled & Grayed" ("Page Enabled State")) -> (s? t:f=w558:T7)
          n309 = property class="Page"(reference=w559, "PageEnb"=w558) -> ()  [unwired: 1 in, 2 out]
        }
        "Error" <- w554
      }
      frame "Stop" {
        n310 = Unbundle By Name(w583) -> ("Parser Queue"=w582:refnum<queue>, "Bus Queue"=w579:refnum<queue>, "Scaling Queue"=w574:refnum<queue>, "Query Queue"=w573:refnum<queue>, "Config Queue"=w565:refnum<queue>)
        n311 = call "ICM Close Sub Panel.vi"("Queue"=w582) -> ("error out"=w580:errorcluster, "Queue Out"=w581:refnum<queue>)  [unwired: 9 in]
        n312 = call "ICM Close Sub Panel.vi"("Queue"=w579) -> ("error out"=w577:errorcluster, "Queue Out"=w578:refnum<queue>)  [unwired: 9 in]
        n313 = call "ICM Close Sub Panel.vi"("Queue"=w574) -> ("error out"=w576:errorcluster, "Queue Out"=w575:refnum<queue>)  [unwired: 9 in]
        n314 = call "ICM Close Sub Panel.vi"("Queue"=w573) -> ("error out"=w571:errorcluster, "Queue Out"=w572:refnum<queue>)  [unwired: 9 in]
        n315 = Release Queue(queue=w581, error in (no error)=w580) -> (error out=w570:errorcluster)  [unwired: 1 in, 2 out]
        n316 = Release Queue(queue=w578, error in (no error)=w577) -> (error out=w569:errorcluster)  [unwired: 1 in, 2 out]
        n317 = Release Queue(queue=w575, error in (no error)=w576) -> (error out=w568:errorcluster)  [unwired: 1 in, 2 out]
        n318 = Release Queue(queue=w572, error in (no error)=w571) -> (error out=w567:errorcluster)  [unwired: 1 in, 2 out]
        n319 = Release Queue(queue=w565) -> (error out=w566:errorcluster)  [unwired: 2 in, 2 out]
        n320 = flat-sequence {
          tunnel: w570 -> [_]
          tunnel: w569 -> [_]
          tunnel: w568 -> [_]
          tunnel: w567 -> [_]
          tunnel: w566 -> [_]
          frame #0 {
          }
        }
        n321 = local write "Tab"(ICM_Editor_Tab."General" ("Tab")) -> ()
        n322 = global write "ICM Editor Stop.vi" "Stop"(FALSE ("Stop")) -> ()
      }
    }
  }
